vi "Store Static VI References for Subpanel.vi"(8 "error in (no error)":errorcluster, 11 "VacuumLines Configuration in":refnum<class "VacuumLines Configuration.lvclass">) -> (0 "error out":errorcluster, 3 "VacuumLines Configuration out":refnum<class "VacuumLines Configuration.lvclass">)   [LabVIEW 2016, in "Hardware.lvlib" / "VacuumLine.lvlib" / "VacuumLines Configuration.lvclass"]
uses:
  <userlib>/Common Components/Hardware/Abstract System/VacuumLine/VacuumLines Configuration/VacuumLines Configuration.lvclass
  <userlib>/Configuration Dialog Actor/Configuration.lvclass
  <userlib>/Common Components/Hardware/Abstract System/VacuumLine/VacuumLine Config/VacuumLine Configuration.lvclass
  <userlib>/Common Components/Hardware/Motor/Motor Config/Motor Configuration.lvclass
  C:/Program Files (x86)/National Instruments/LabVIEW 2016/user.lib/Configuration Dialog Actor/Configuration.lvclass
  <userlib>/Common Components/UserPwd DB/UserPwd DB Config/UserPwd DB Configuration.lvclass
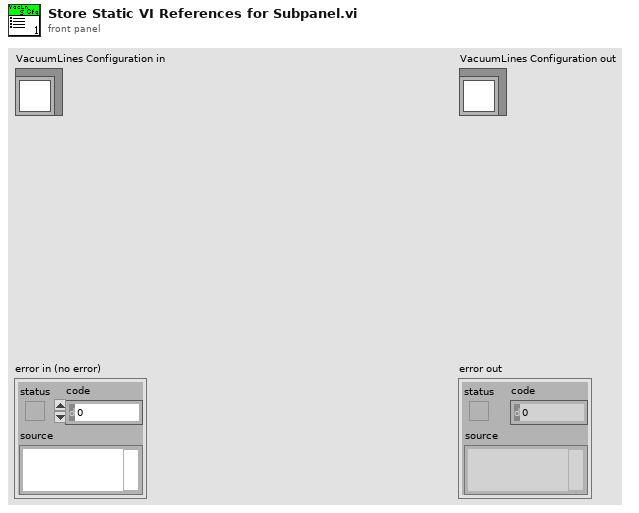
[diagram p1: front panel]
types:
  T1 = typedef "Configuration.lvlib/Configuration.lvclass/Data Retrieved by Lookup Table.ctl" = cluster{"VI Refnum":refnum<vi>, "Help Text":string}
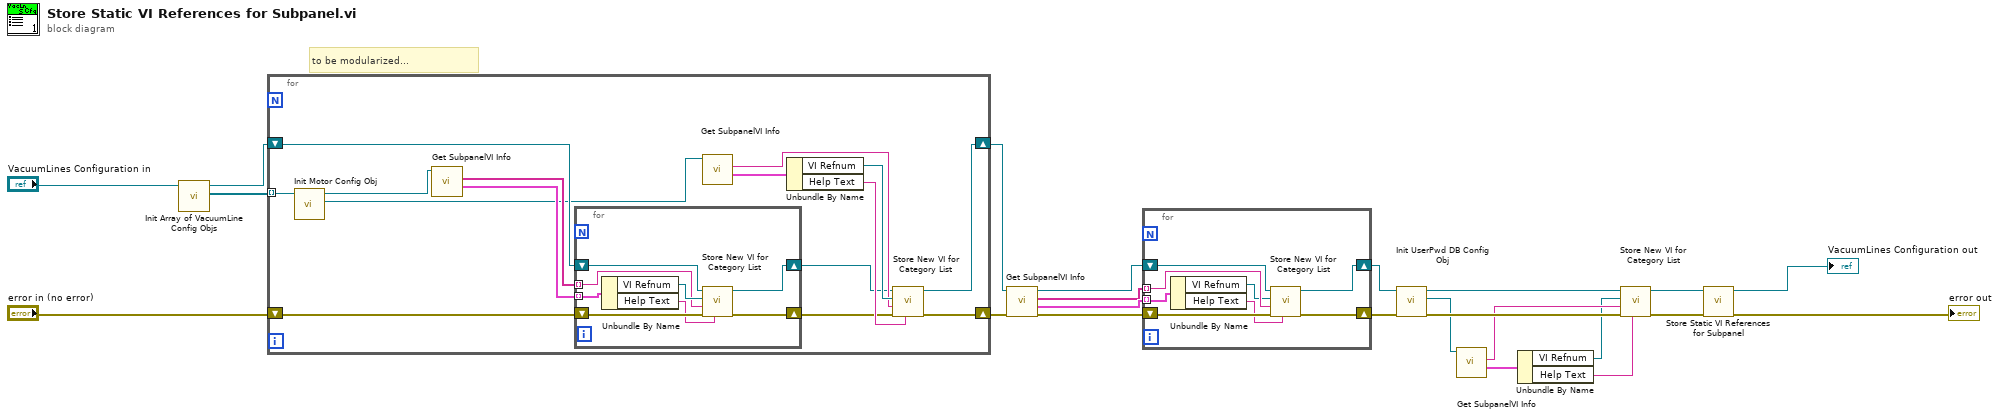
[diagram p0: block diagram]
diagram:
  # "to be modularized..."
  n1 = call <userlib>:"Init Array of VacuumLine Config Objs.vi"("VacuumLines Configuration in"="VacuumLines Configuration in") -> ("Array of VacuumLine Config Objs"=w18:refnum<class "VacuumLine Configuration.lvclass">[], "VacuumLines Configuration out"=w19:refnum<class "VacuumLines Configuration.lvclass">)  [unwired: 8 in, 1 out]
  n2 = for {
    tunnel: w18 -> [w32] mode=indexing
    shift-right: [w33] -> w22
    shift-left: "error in (no error)" -> [w31]
    shift-right: [w30] -> w16
    shift-left: w19 -> [w28]
    n3 = call <userlib>:"Init Motor Config Obj.vi"("VacuumLine Configuration in"=w32) -> ("Motor Config Obj"=w24:refnum<class "Motor Configuration.lvclass">, "VacuumLine Configuration out"=w37:refnum<class "VacuumLine Configuration.lvclass">)  [unwired: 8 in, 1 out]
    n4 = call-dynamic "Get SubpanelVI Info.vi"("VacuumLine Configuration in"=w37) -> ("Array of Subpanel VI data"=w26:T1[], "Array of Category string"=w25:string[])  [unwired: 7 in, 2 out]
    n5 = for {
      tunnel: w26 -> [w42] mode=indexing
      tunnel: w25 -> [w40] mode=indexing
      shift-right: [w45] -> w29
      shift-left: w31 -> [w46]
      shift-right: [w43] -> w27
      shift-left: w28 -> [w44]
      n6 = Unbundle By Name(w42) -> ("VI Refnum"=w41:refnum<vi>, "Help Text"=w39:string)
      n7 = call <userlib>:"Store New VI for Category List.vi"("Help Text"=w39, "error in (no error)"=w46, "String"=w40, "VI Refnum"=w41, "Configuration in"=w44) -> ("error out"=w45:errorcluster, "Configuration out"=w43:refnum<class "VacuumLines Configuration.lvclass">)  [unwired: 5 in]
    }
    n8 = call-dynamic "Get SubpanelVI Info.vi"("Motor Configuration in"=w24) -> ("Subpanel VI data"=w38:T1, "Category string"=w34:string)  [unwired: 7 in, 2 out]
    n9 = Unbundle By Name(w38) -> ("VI Refnum"=w36:refnum<vi>, "Help Text"=w35:string)
    n10 = call <userlib>:"Store New VI for Category List.vi"("Help Text"=w35, "error in (no error)"=w29, "String"=w34, "VI Refnum"=w36, "Configuration in"=w27) -> ("error out"=w33:errorcluster, "Configuration out"=w30:refnum<class "VacuumLines Configuration.lvclass">)  [unwired: 5 in]
  }
  n11 = call-dynamic "Get SubpanelVI Info.vi"("error in (no error)"=w22, "VacuumLines Configuration in"=w16) -> ("error out"=w17:errorcluster, "Array of Subpanel VI data"=w14:T1[], "Array of Category string"=w13:string[], "VacuumLines Configuration out"=w15:refnum<class "VacuumLines Configuration.lvclass">)  [unwired: 6 in]
  n12 = for {
    tunnel: w14 -> [w50] mode=indexing
    shift-right: [w53] -> w11
    shift-left: w17 -> [w54]
    shift-right: [w51] -> w9
    shift-left: w15 -> [w52]
    tunnel: w13 -> [w49] mode=indexing
    n13 = Unbundle By Name(w50) -> ("VI Refnum"=w48:refnum<vi>, "Help Text"=w47:string)
    n14 = call <userlib>:"Store New VI for Category List.vi"("Help Text"=w47, "error in (no error)"=w54, "String"=w49, "VI Refnum"=w48, "Configuration in"=w52) -> ("error out"=w53:errorcluster, "Configuration out"=w51:refnum<class "VacuumLines Configuration.lvclass">)  [unwired: 5 in]
  }
  n15 = call <userlib>:"Init UserPwd DB Config Obj.vi"("error in (no error)"=w11, "VacuumLines Configuration in"=w9) -> ("error out"=w10:errorcluster, "UserPwd DB Configuration Obj"=w8:refnum<class "UserPwd DB Configuration.lvclass">, "VacuumLines Configuration out"=w6:refnum<class "VacuumLines Configuration.lvclass">)  [unwired: 7 in]
  n16 = call-dynamic "Get SubpanelVI Info.vi"("Configuration in"=w8) -> ("Subpanel VI data"=w3:T1, "Category string"=w4:string)  [unwired: 7 in, 2 out]
  n17 = Unbundle By Name(w3) -> ("VI Refnum"=w2:refnum<vi>, "Help Text"=w1:string)
  n18 = call <userlib>:"Store New VI for Category List.vi"("Help Text"=w1, "error in (no error)"=w10, "String"=w4, "VI Refnum"=w2, "Configuration in"=w6) -> ("error out"=w7:errorcluster, "Configuration out"=w5:refnum<class "VacuumLines Configuration.lvclass">)  [unwired: 5 in]
  n19 = call-parent "Store Static VI References for Subpanel.vi"("error in (no error)"=w7, "Configuration in"=w5) -> ("error out"=→"error out":errorcluster, "Configuration out"=→"VacuumLines Configuration out":refnum<class "VacuumLines Configuration.lvclass">)  [unwired: 8 in]
